vi "Default Instrument Setup.vi"(8 "error in (no error)":errorcluster, 11 "VISA resource name":refnum<visa-resource-name>) -> (0 "error out":errorcluster, 3 "VISA resource name out":refnum<visa-resource-name>)   [LabVIEW 2018, in "JULABO DeviceDriver.lvlib"]
doc: "This Utility VI sends a default command string to the instrument whenever a new VISA session is opened, or the instrument is reset. This VI is used as a subVI for the <B>Initialize</B> and <B>Reset</B> VIs. Altering this VI could cause these two VIs to operate incorrectly."
uses:
  JULABO DeviceDriver.lvlib
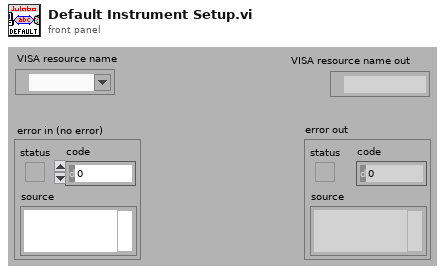
[diagram p1: front panel]
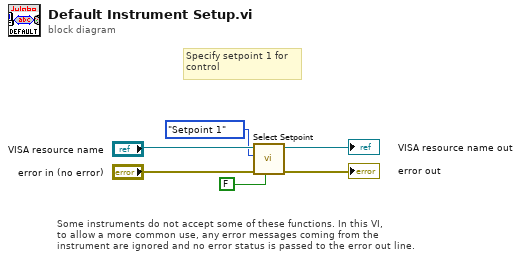
[diagram p0: block diagram]
diagram:
  # "Some instruments do not accept some of these functions. In this VI,\nto allow a more common use, any error messages coming from the\ninstrument are ignored and no error status is passed to the error out line."
  # "Specify setpoint 1 for \ncontrol"
  n1 = call "Select Setpoint.vi"("parseError? T:Yes"=FALSE, "error in (no error)"="error in (no error)", "Setpoint (Setpoint1: Default)"=enum16{"Setpoint 1", "Setpoint 2", "Setpoint 3"}."Setpoint 1" ("Setpoint"), "VISA resource name"="VISA resource name") -> ("error out"=→"error out":errorcluster, "VISA resource name out"=→"VISA resource name out":refnum<visa-resource-name>)  [unwired: 6 in]
